vi "Multiple Roots Visualization.vi"() -> ()   [LabVIEW 2020, in "NI_VIAnCFGDataStructure.lvlib" / "Tree.lvclass"]
uses:
  <vilib>/addons/analyzer/VIAnCFGDataStructure/Tree Manager/Tree.lvclass
panel:
  out "All Names":string[](array[string])=["Child 3", "Parent 1", "Child 2", "Parent 2", "Child 1"]
  out "All IDs":string[](array[string])=["GDyiH8xC8K2eXxAD", "J1GTkAhb8Y8anQWl", "fRClFkPRThmhJCCu", "h2yLWdqAgvQAAIFp", "mh36Ej5eWly8kXuV"]
  out "Roots Names":string[](array[string])=["Parent 1", "Parent 2"]
  out "Roots IDs":string[](array[string])=["J1GTkAhb8Y8anQWl", "h2yLWdqAgvQAAIFp"]
  in  "Tree 2":string(tree)
  in  "Tree":string(tree)
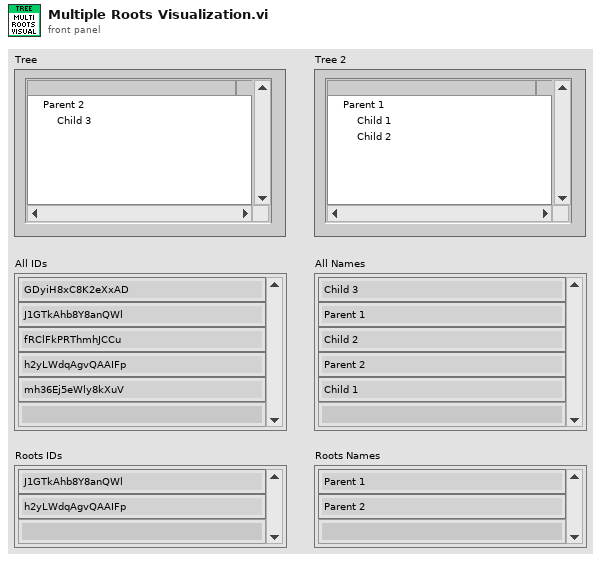
[diagram p1: front panel]
types:
  T1 = typedef "NI_VIAnCFGDataStructure.lvlib/Tree.lvclass/Session Handle.ctl" = refnum<data-value>
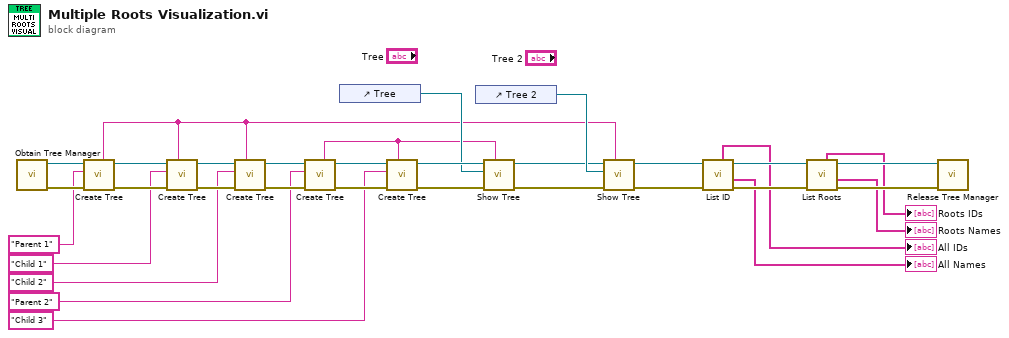
[diagram p0: block diagram]
diagram:
  n1 = call <vilib>:"Obtain Tree Manager.vi"() -> ("Error Out"=w32:errorcluster, "Tree"=w33:T1)  [unwired: 10 in]
  n2 = call <vilib>:"Create Tree.vi"("Error In"=w32, "Name"="Parent 1", "Tree Manager"=w33) -> ("Error Out"=w30:errorcluster, "Tree Manager"=w31:T1, "Unique ID"=w1:string)  [unwired: 6 in]
  n3 = call <vilib>:"Create Tree.vi"("Parent ID (empty)"=w1, "Error In"=w30, "Name"="Child 1", "Tree Manager"=w31) -> ("Error Out"=w28:errorcluster, "Tree Manager"=w29:T1)  [unwired: 5 in, 1 out]
  n4 = call <vilib>:"Create Tree.vi"("Parent ID (empty)"=w1, "Error In"=w28, "Name"="Child 2", "Tree Manager"=w29) -> ("Error Out"=w26:errorcluster, "Tree Manager"=w27:T1)  [unwired: 5 in, 1 out]
  n5 = call <vilib>:"Create Tree.vi"("Error In"=w26, "Name"="Parent 2", "Tree Manager"=w27) -> ("Error Out"=w24:errorcluster, "Tree Manager"=w25:T1, "Unique ID"=w6:string)  [unwired: 6 in]
  n6 = control-ref of="Tree"() -> (w16:refnum<vi>)
  n7 = call <vilib>:"Create Tree.vi"("Parent ID (empty)"=w6, "Error In"=w24, "Name"="Child 3", "Tree Manager"=w25) -> ("Error Out"=w22:errorcluster, "Tree Manager"=w23:T1)  [unwired: 5 in, 1 out]
  n8 = control-ref of="Tree 2"() -> (w17:refnum<vi>)
  n9 = call <vilib>:"Show Tree.vi"("Root ID"=w6, "Error In"=w22, "Tree Ref"=w16, "Tree"=w23) -> ("Error Out"=w12:errorcluster, "Tree"=w13:T1)  [unwired: 6 in]
  n10 = call <vilib>:"Show Tree.vi"("Root ID"=w1, "Error In"=w12, "Tree Ref"=w17, "Tree"=w13) -> ("Error Out"=w8:errorcluster, "Tree"=w11:T1)  [unwired: 6 in]
  n11 = call <vilib>:"List ID.vi"("Error In"=w8, "Tree Manager"=w11) -> ("Error Out"=w9:errorcluster, "Child Names"=→"All Names":string[], "Tree Manager"=w10:T1, "Child IDs"=→"All IDs":string[])  [unwired: 6 in]
  n12 = call <vilib>:"List Roots.vi"("Error In"=w9, "Tree"=w10) -> ("Error Out"=w15:errorcluster, "Roots Names"=→"Roots Names":string[], "Tree"=w14:T1, "Roots IDs"=→"Roots IDs":string[])  [unwired: 6 in]
  n13 = call <vilib>:"Release Tree Manager.vi"("Error In"=w15, "Tree"=w14) -> ()  [unwired: 9 in, 1 out]
